vi "display_lucky_num.vi"(0 "Name":string caption="Enter your name", 5 "Birthday":timestamp caption="Select Birthday" format="%<%x>T", 11 "error in":errorcluster) -> (4 "lucky_num":i32, 6 "Back 2":T1, 8 "path":path, 15 "error out":errorcluster)   [LabVIEW 2023]
doc: "Display the lucky number of the user."
uses:
  custom_elements/continue.ctl
  custom_elements/back_button.ctl
panel:
  in  "Back":T1
  out "lucky_num_text":string
  in  "stop":T2
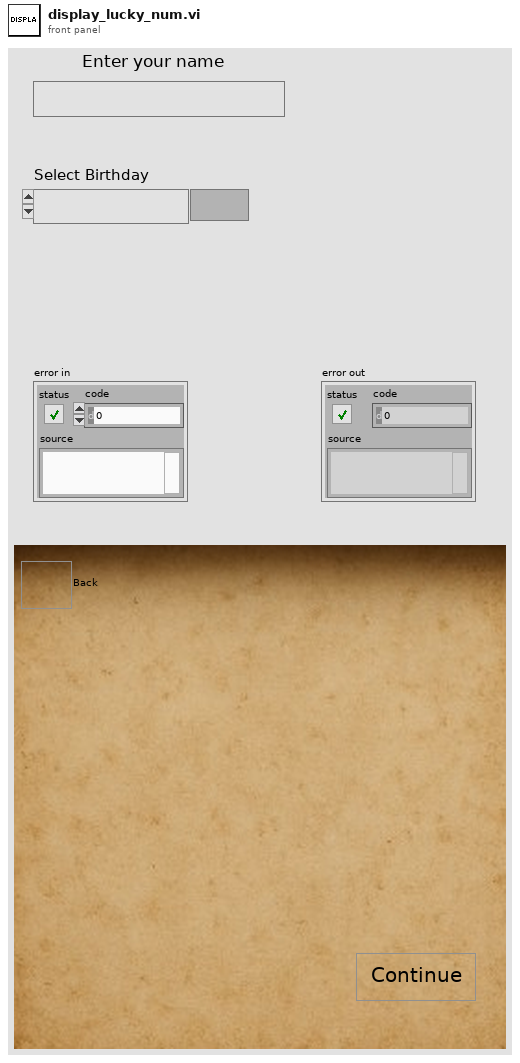
[diagram p1: front panel]
types:
  T1 = typedef "back_button.ctl" = bool
  T2 = typedef "continue.ctl" = bool
  T3 = typedef "LVDateTimeRec.ctl" = cluster{"fractional second":dbl, "second":i32, "minute":i32, "hour":i32, "day of month":i32, "month":i32, "year":i32, "day of week":i32, "day of year":i32, "DST":i32}
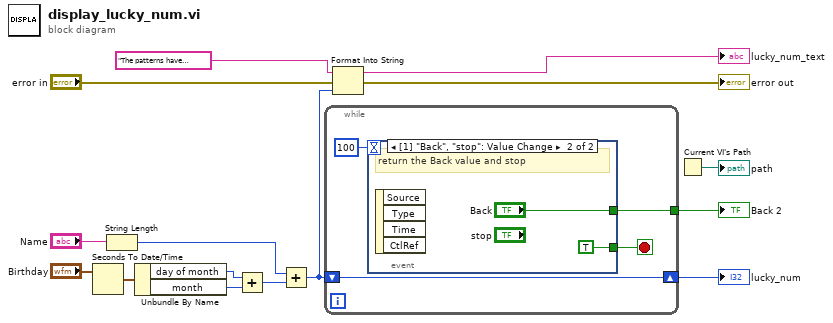
[diagram p0: block diagram]
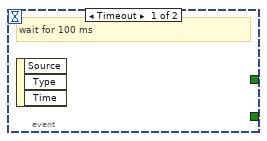
[diagram p2: hidden frame]
diagram:
  n1 = Seconds To Date/Time(time stamp (now)="Birthday") -> (date time rec=w12:T3)  [unwired: 1 in]
  n2 = String Length(string="Name") -> (length=w9:i32)
  n3 = Unbundle By Name(w12) -> ("day of month"=w11:i32, "month"=w10:i32)
  n4 = Add(x=w11, y=w10) -> (x+y=w8:i32)
  n5 = Add(x=w9, y=w8) -> (x+y=w6:i32)
  n6 = while {
    shift-right: [w19] -> w7
    shift-left: w6 -> [w19]
    tunnel: [w17] -> w1
    stop <- w18 stop-if-true
    n7 = event shown="[1] \"Back\", \"stop\": Value Change" {
      selector: _ -> [_ _]
      dyn-events: _ -> [_ _]
      timeout: 100 -> [_ _]
      tunnel: [_ TRUE] -> w18
      tunnel: [_ "Back"] -> w17
      event Timeout {
        # "wait for 100 ms"
        n8 = event-data() -> ()  [unwired: 1 in, 3 out]
      }
      event Value Change {
        # "return the Back value and stop"
        n9 = event-data() -> ()  [unwired: 1 in, 4 out]
      }
    }
  }
  "lucky_num" <- w7
  "Back 2" <- w1
  n10 = Format Into String(initial string="The patterns have aligned, seeker. From the great loom where destinies are spun, a singular vibration emerges, a number meant for thee alone...Hark! The Digit that resonates with the core of thy being, the very Number that whispers of thy hidden potential, is...", error in="error in", w6) -> (resulting string=→"lucky_num_text":string, error out=→"error out":errorcluster)  [unwired: 1 in]
  n11 = Current VI's Path() -> (path=→"path":path)
